vi "Linear Helicopter Controller.vi"(4 "travel speed (deg/sec)":dbl, 5 "Elevation Setpoint":dbl(slide)=14.285714285714286 scale=0.0..20.0 scale format="%.2f", 6 "pitch speed (deg/sec)":dbl, 7 "Travel Setpoint":dbl(knob)=14.222946670967534 scale=-180.0..180.0, 8 "elevation speed (deg/sec)":dbl, 9 "travel angle (deg)":dbl, 10 "pitch angle (deg)":dbl, 11 "elevation angle (deg)":dbl) -> (2 "motor voltage 2":dbl, 3 "motor voltage 1":dbl)   [LabVIEW 2014]
uses:
  Helicopter SubVIs/cdex_Elevation PID.vi
  Helicopter SubVIs/cdex_Pitch PID.vi
  Helicopter SubVIs/cdex_Position PID.vi
  <vilib>/Simulation/Implementation/Shared/SIMSCR Execution Mode.ctl
  <vilib>/Simulation/Scripting/Companion Diagram/SimConfigNode/SimParams.ctl
  <vilib>/Simulation/Scripting/Companion Diagram/SimConfigNode/_simSolvers.ctl
  <vilib>/Simulation/Param Hierarchy/Typedefs/SIMPH Param Control Actions.ctl
  <vilib>/Simulation/Implementation/Shared/NILVSim_ParamChanged.vi
  <vilib>/Simulation/Implementation/Shared/NILVSIM_BeginStep.vi
  <vilib>/Simulation/SignalArithmetic/Implementation/NILVSim Gain.llb/SIM Gain (scalar).vi
  <vilib>/Simulation/Implementation/Shared/NILVSim_Manager.vi
  <vilib>/Utility/error.llb/Clear Errors.vi
  <vilib>/Simulation/Implementation/Shared/NILVSim_FinalizeModel.vi
  <vilib>/Simulation/Implementation/Shared/SIM Unbundle Sim Info.vi
  <vilib>/Simulation/Implementation/Shared/SIMSH Read Queue.vi
  <vilib>/Simulation/Implementation/Shared/NILVSim_Initialize.vi
  <vilib>/Simulation/Utility/Implementation/NILVSim Get Time and IsAcceptedStep.vi
  <vilib>/Simulation/Implementation/Shared/NILVSim_GetModelError.vi
  <vilib>/Simulation/Implementation/Shared/SIM SimErrorHandler.vi
  <vilib>/Simulation/Implementation/Shared/SIM Bundle Sim Info.vi
  <vilib>/Simulation/Scripting/Companion Diagram/SimConfigNode/SimDog.xnode
  <vilib>/Simulation/Implementation/XNodeFramework/SimXNode/SimX.xnode
  <vilib>/Simulation/Implementation/Shared/NI_SIM_Implementation.lvlib
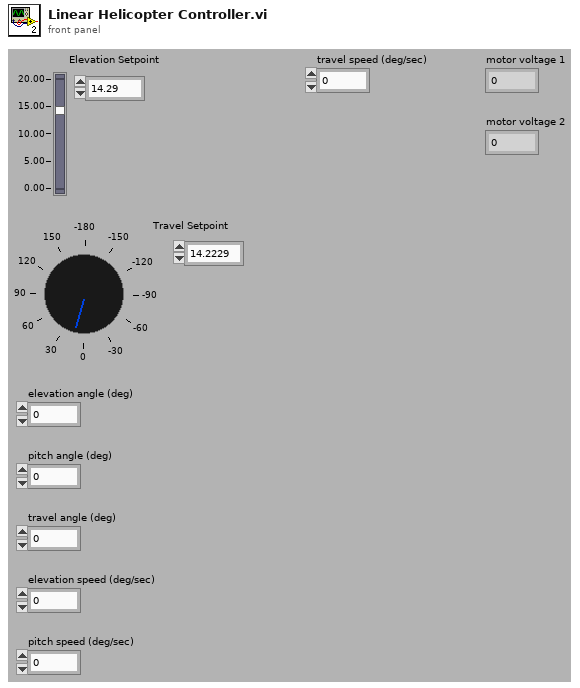
[diagram p1: front panel]
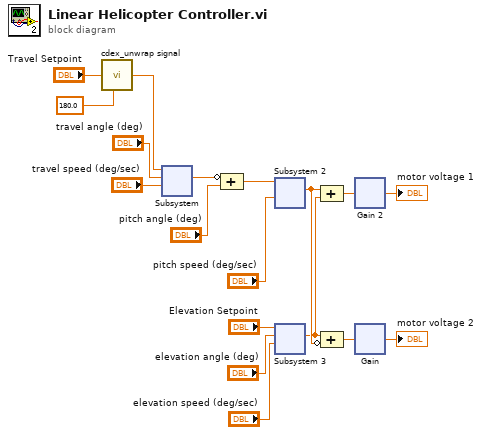
[diagram p0: block diagram]
diagram:
  n1 = call "cdex_unwrap signal.vi"("input"="Travel Setpoint", "wrap range"=180.0) -> ("output"=w16:dbl)  [unwired: 7 in]
  n2 = xnode ("Subsystem")("travel speed"="travel speed (deg/sec)", "travel angle"="travel angle (deg)", "travel set point"=w16) -> ("Output (u)"=w10:dbl)  [unwired: 8 out]
  n3 = Compound Arithmetic op=ADD ("Compound Arithmetic 3")(invert w10, "pitch angle (deg)") -> (w8:dbl)
  n4 = xnode ("Subsystem 2")("pitch speed"="pitch speed (deg/sec)", "pitch set point"=w8) -> ("Output (u)"=w9:dbl)  [unwired: 9 out]
  n5 = xnode ("Subsystem 3")("elevation speed"="elevation speed (deg/sec)", "elevation angle"="elevation angle (deg)", "elevation set point"="Elevation Setpoint") -> ("Output (u)"=w7:dbl)  [unwired: 8 out]
  n6 = Compound Arithmetic op=unknown(w9, w7) -> (w12:dbl)
  n7 = Compound Arithmetic op=unknown ("Compound Arithmetic 2")(w7, invert w9) -> (w11:dbl)
  n8 = xnode ("Gain 2")("input"=w12) -> ("output"=→"motor voltage 1":dbl)  [unwired: 3 in]
  n9 = xnode ("Gain")("input"=w11) -> ("output"=→"motor voltage 2":dbl)  [unwired: 3 in]
